vi "NF LI56xx dvr Initialize.vi"(8 "error in (no error)":errorcluster caption="Error IN", 9 "isReset":bool, 10 "isIdQuery":bool=TRUE, 11 "VISA resource name":refnum<visa-resource-name>="GPIB0::2::INSTR") -> (0 "error out":errorcluster caption="Error OUT", 2 "type":string, 3 "VISA resource name out":refnum<visa-resource-name>)   [LabVIEW 2019]
doc: "open the interface of instrument."
uses:
  <vilib>/regexp/Match Regular Expression.xnode
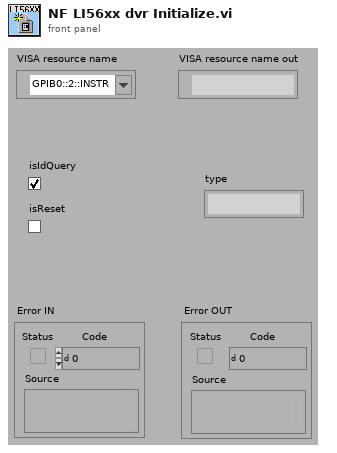
[diagram p1: front panel]
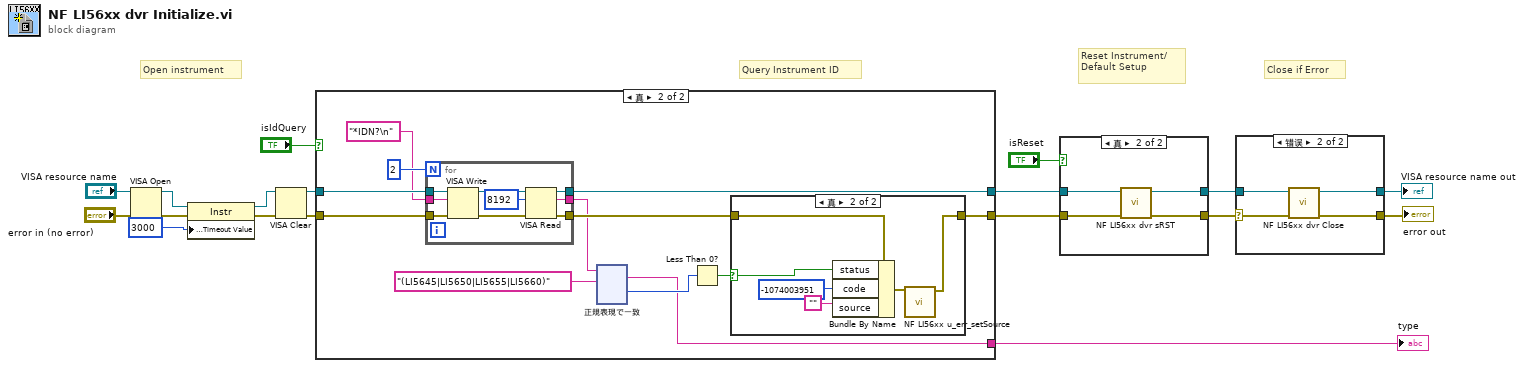
[diagram p0: block diagram]
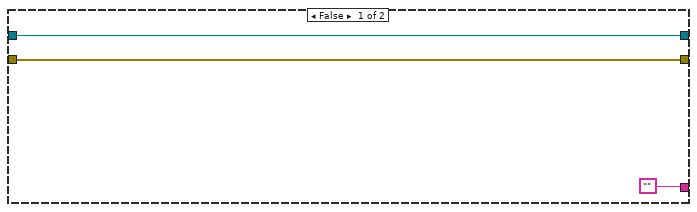
[diagram p2: hidden frame]
diagram:
  # "Close if Error"
  # "Query Instrument ID"
  # "Reset Instrument/\nDefault Setup"
  # "Open instrument"
  n1 = VISA Open(error in (no error)="error in (no error)", VISA resource name="VISA resource name") -> (VISA resource name=w5:refnum<visa-resource-name>, error out=w4:errorcluster)  [unwired: 3 in]
  n2 = property class="Instr"(reference=w5, error in=w4, "General Settings:Timeout Value"=u32 3000) -> (reference out=w7:refnum<visa-resource-name>, error out=w10:errorcluster)
  n3 = VISA Clear(VISA resource name=w7, error in (no error)=w10) -> (VISA resource name out=w8:refnum<visa-resource-name>, error out=w9:errorcluster)
  n4 = case shown="真" "isIdQuery" {
    tunnel: w9 -> [w20 w28]
    tunnel: w8 -> [w21 w29]
    tunnel: [w21 w31] -> w16
    tunnel: [w20 w33] -> w15
    tunnel: ["" w22] -> w1
    frame False {
    }
    frame True {
      n5 = for {
        N: 2 -> [_]
        tunnel: [w151] -> w31
        tunnel: [w150] -> w30
        tunnel: w29 -> [w149]
        tunnel: w28 -> [w148]
        tunnel: "*IDN?\n" ("³K\\»") -> [w147]
        tunnel: [w146] -> w23
        n6 = VISA Write(VISA resource name=w149, write buffer=w147, error in (no error)=w148) -> (VISA resource name out=w153:refnum<visa-resource-name>, error out=w152:errorcluster)  [unwired: 1 out]
        n7 = VISA Read(VISA resource name=w153, byte count=u32 8192 ("バイトカウント"), error in (no error)=w152) -> (VISA resource name out=w151:refnum<visa-resource-name>, read buffer=w146:string, error out=w150:errorcluster)  [unwired: 1 out]
      }
      n8 = xnode "正規表現で一致"("“ü—Í•¶Žš—ñ"=w23, "³K\\»"="(LI5645|LI5650|LI5655|LI5660)" ("³K\\»")) -> ("‘S‘Ìˆê’v"=w22:string, "一致後オフセット"=w25:i32)  [unwired: 4 in, 3 out]
      n9 = Less Than 0?(x=w25) -> (x < 0?=w32:bool)
      n10 = case shown="真" w32 {
        selector: w32 -> [_ w158]
        tunnel: w30 -> [w154 w160]
        tunnel: [w154 w155] -> w33
        frame False {
        }
        frame True {
          n11 = Bundle By Name(cluster=w160, "status"=w158, "code"=-1074003951, "source"="") -> (w156:errorcluster)
          n12 = call "NF LI56xx u_err_setSource.vi"("error in (no error)"=w156) -> ("error out"=w155:errorcluster)  [unwired: 10 in]
        }
      }
    }
  }
  "type" <- w1
  n13 = case shown="真" "isReset" {
    tunnel: w16 -> [w162 w166]
    tunnel: w15 -> [w161 w163]
    tunnel: [w162 w165] -> w14
    tunnel: [w161 w164] -> w13
    frame False {
    }
    frame True {
      n14 = call "NF LI56xx dvr sRST.vi"("error in"=w163, "VISA resource name"=w166) -> ("error out"=w164:errorcluster, "VISA resource name copy"=w165:refnum<visa-resource-name>)  [unwired: 8 in]
    }
  }
  n15 = case shown="错误" w13 {
    selector: w13 -> [w168 w169]
    tunnel: [w168 w170] -> w2
    tunnel: w14 -> [w167 w172]
    tunnel: [w167 w171] -> w18
    frame No Error {
    }
    frame Error {
      n16 = call "NF LI56xx dvr Close.vi"("error in (no error)"=w169, "VISA resource name"=w172) -> ("error out"=w170:errorcluster, "VISA resource name out"=w171:refnum<visa-resource-name>)  [unwired: 8 in]
    }
  }
  "VISA resource name out" <- w18
  "error out" <- w2
